vi "Error Test Transmit Period.vi"(6 "error text in":string, 8 "error in":errorcluster, 10 "transmit period":u32) -> (0 "error out":errorcluster)   [LabVIEW 2020]
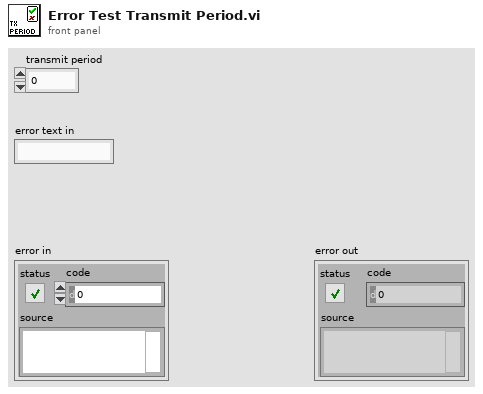
[diagram p1: front panel]
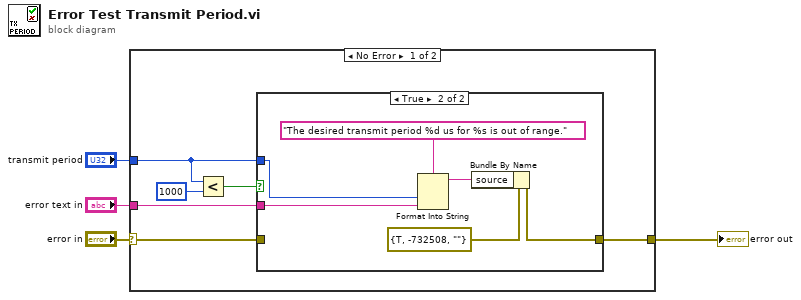
[diagram p0: block diagram]
diagram:
  n1 = case shown="No Error" "error in" {
    selector: "error in" -> [w10 w18]
    tunnel: [w9 w18] -> w3
    tunnel: "transmit period" -> [w5 _]
    tunnel: "error text in" -> [w8 _]
    frame No Error {
      n2 = Less?(x=w5, y=u32 1000) -> (x < y?=w6:bool)
      n3 = case shown="True" w6 {
        tunnel: w10 -> [w11 _]
        tunnel: [w11 w15] -> w9
        tunnel: w8 -> [_ w13]
        tunnel: w5 -> [_ w12]
        frame False {
        }
        frame True {
          n4 = Format Into String(format string="The desired transmit period %d us for %s is out of range." ("source"), w12, w13) -> (resulting string=w17:string)  [unwired: 2 in, 1 out]
          n5 = Bundle By Name(cluster=errorcluster {"status"=TRUE, "code"=-732508, "source"=""} ("error constant"), "source"=w17) -> (w15:errorcluster)
        }
      }
    }
    frame Error {
    }
  }
  "error out" <- w3
